vi "MenuSelection Response.vi"(6 "Coords":T1, 8 "error in (no error)":errorcluster, 9 "Menu Name":string, 10 "Menu Tag":string, 11 "Editor Handler in":refnum<class "Handler 4.lvclass">) -> (0 "error out":errorcluster, 3 "Editor Handler out":refnum<class "Handler 4.lvclass">)   [LabVIEW 2017, in "Handler 4.lvclass"]
uses:
  Handler 4.lvclass
  <vilib>/Utility/miscctls.llb/LVPoint32TypeDef.ctl
  <vilib>/LIEF/Image Editor Handler/Image Editor Handler.lvclass
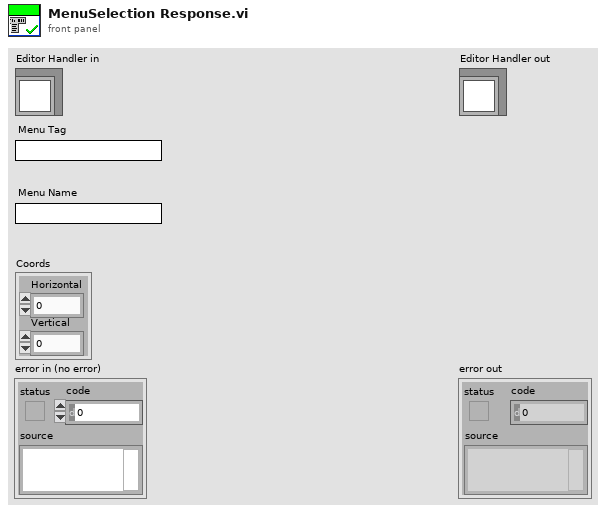
[diagram p1: front panel]
types:
  T1 = typedef "LVPoint32TypeDef.ctl" = cluster{"Horizontal":i32, "Vertical":i32}
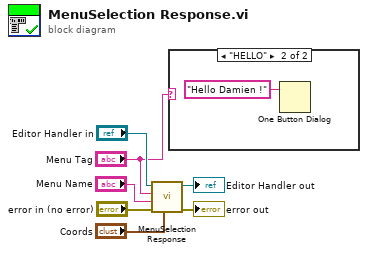
[diagram p0: block diagram]
diagram:
  n1 = call-parent "MenuSelection Response.vi"("Coords"="Coords", "error in (no error)"="error in (no error)", "Menu Name"="Menu Name", "Menu Tag"="Menu Tag", "Editor Handler in"="Editor Handler in") -> ("error out"=→"error out":errorcluster, "Editor Handler out"=→"Editor Handler out":refnum<class "Handler 4.lvclass">)  [unwired: 5 in]
  n2 = case shown="\"HELLO\"" "Menu Tag" {
    frame "False", Default {
    }
    frame "HELLO" {
      n3 = One Button Dialog(message="Hello Damien !") -> ()  [unwired: 1 in, 1 out]
    }
  }
